vi "LS336_read_temp - Copy.vi"(6 "Data Source (0:Kelvin)":u16(ring) items=["Kelvin", "Celsius", "Sensor Units"], 10 "Input I(0:A)":u16(ring) items=["A", "B", "C", "D"], 11 "VISA Refnum in":refnum<visa-resource-name>) -> (3 "Sensor Data":dbl)   [LabVIEW 2017]
uses:
  <instrlib>/Lake Shore 336/Public/Data/Sensor Data (Single Reading).vi
  <vilib>/Utility/file.llb/Write Delimited Spreadsheet (DBL).vi
  <instrlib>/Lake Shore 336/Lake Shore 336.lvlib
panel:
  in  "milliseconds to wait":u32=60000
  out "Sensor Data 2":dbl
  in  "Input II (0:A) 2":u16(ring) items=["A", "B", "C", "D"]
  in  "file path (dialog if empty)":path
  in  "Stop Button":bool
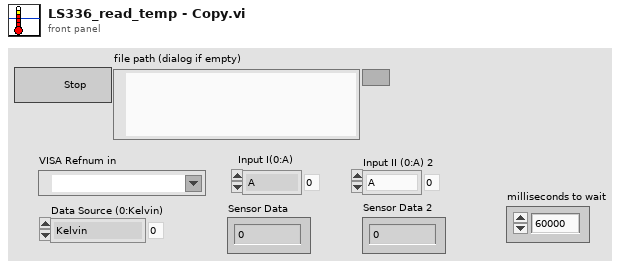
[diagram p1: front panel]
types:
  T1 = cluster{"Baud Rate":u32, "Parity":u16, "Data Bits":u16, "Stop Bits":u16, "Flow Control":u16}
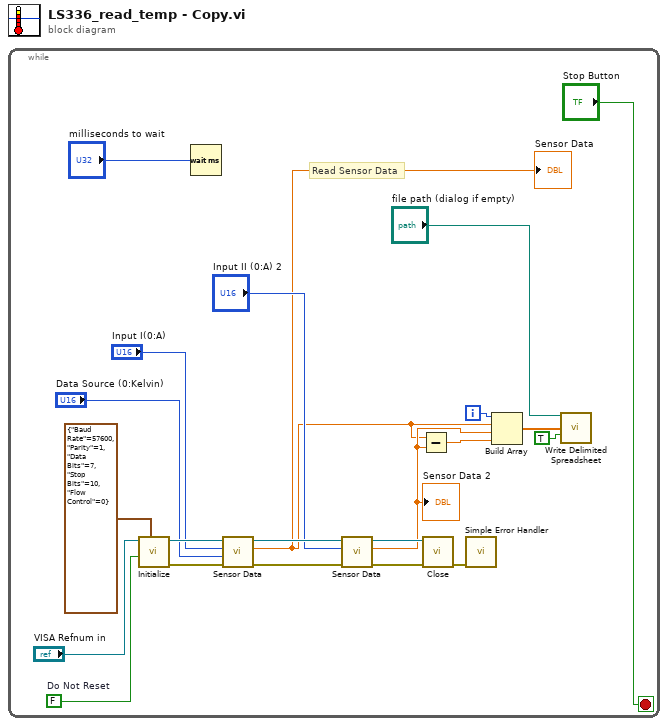
[diagram p0: block diagram]
diagram:
  n1 = while {
    i -> [w9]
    stop <- "Stop Button" stop-if-true
    w17 = FALSE  # Do Not Reset
    # "Read Sensor Data"
    n2 = call <instrlib>:"Initialize.vi"("Serial Configuration"=T1 {"Baud Rate"=57600, "Parity"=1, "Data Bits"=7, "Stop Bits"=10, "Flow Control"=0}, "Reset (True)"=w17, "VISA resource name"="VISA Refnum in") -> ("error out"=w22:errorcluster, "VISA resource name out"=w21:refnum<visa-resource-name>)  [unwired: 7 in]
    n3 = Wait (ms)(milliseconds to wait="milliseconds to wait") -> ()  [unwired: 1 out]
    n4 = call-poly <instrlib>:"Sensor Data.vi"("error in (no error)"=w22, "Data Source (0:Kelvin)"="Data Source (0:Kelvin)", "Input (0:A)"="Input I(0:A)", "VISA resource name"=w21) -> ("error out"=w6:errorcluster, "Sensor Data"=w1:dbl, "VISA resource name out"=w8:refnum<visa-resource-name>)  [unwired: 5 in]
    "Sensor Data" <- w1
    n5 = call-poly <instrlib>:"Sensor Data.vi"("error in (no error)"=w6, "Input (0:A)"="Input II (0:A) 2", "VISA resource name"=w8) -> ("error out"=w5:errorcluster, "Sensor Data"=w2:dbl, "VISA resource name out"=w7:refnum<visa-resource-name>)  [unwired: 6 in]
    "Sensor Data 2" <- w2
    n6 = Subtract(x=w1, y=w2) -> (x-y=w3:dbl)
    n7 = call <instrlib>:"Close.vi"("error in (no error)"=w5, "VISA resource name"=w7) -> ("error out"=w16:errorcluster)  [unwired: 9 in]
    n8 = call <vilib>:"Simple Error Handler.vi"("error in (no error)"=w16) -> ()  [unwired: 4 in, 5 out]
    n9 = Build Array(w9, w1, w2, w3) -> (w11:dbl[])
    n10 = call-poly <vilib>:"Write Delimited Spreadsheet.vi"("file path (dialog if empty)"="file path (dialog if empty)", "1D data"=w11, "append to file? (new file:F)"=TRUE) -> ()  [unwired: 11 in, 2 out]
  }
